vi "PixieReadGDT.vi"(8 "error in (no error)":errorcluster, 10 "ChanNum":u16) -> (0 "error out":errorcluster, 2 "GDT":dbl)   [LabVIEW 2013]
doc: "Use this template to build a VI to use as a subVI."
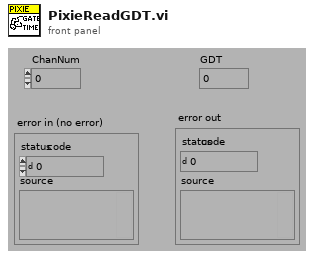
[diagram p1: front panel]
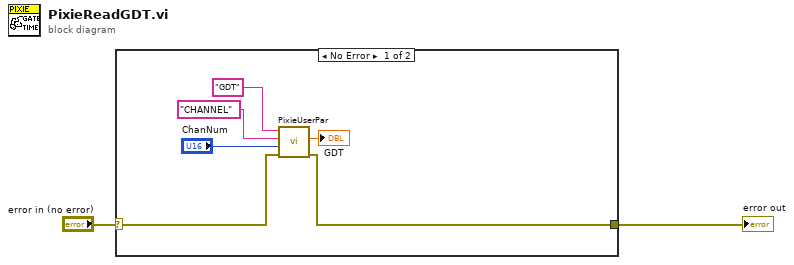
[diagram p0: block diagram]
diagram:
  n1 = case shown="No Error" "error in (no error)" {
    selector: "error in (no error)" -> [w5 w9]
    tunnel: [w6 w9] -> w1
    frame No Error {
      n2 = call "PixieUserPar.vi"("error in (no error)"=w5, "ChanNum"="ChanNum", "User_Par_Type"="CHANNEL", "User_Par_Name"="GDT") -> ("error out"=w6:errorcluster, "User_Par_Value"=→"GDT":dbl)  [unwired: 1 in, 5 out]
    }
    frame Error {
    }
  }
  "error out" <- w1
